vi "CALC_MARK_FUNC_SEL.vi"(0 "VISA IN":refnum<visa-resource-name>, 1 "Marker number":i32=1, 2 "Function":string(combo)="MAX", 5 "error in":errorcluster, 7 "Channel":i32=1) -> (14 "VISA Out":refnum<visa-resource-name>, 19 "error out":errorcluster)   [LabVIEW 2018, in "PNA-X.lvlib"]
doc: "CALCulate<cnum>:MARKer<mkr>:FUNCtion[:SELect] <char> \n(Read-Write) Sets the search function that the specified marker will perform when executed. To \nexecute (or perform) the function, use: \nCALC:MARK:FUNC:EXEC or \nCALC:MARK:FUNC:TRAC ON to automatically execute the search every sweep. \nSee Critical Note \nParameters \n<cnum> Channel number of the measurement. There must be a selected measurement on \nthat channel. If unspecified, <cnum> is set to 1. \n<mkr> Any marker number from 1 to 10; if unspecified, value is set to 1. \n<char> Marker function. Choose from: \nMAXimum - finds the highest value \nMINimum - finds the lowest value \nRPEak - finds the next valid peak to the right \nLPEak - finds the next valid peak to the left \nNPEak - finds the next highest value among the valid peaks \nTARGet - finds the target value to the right, wraps around to the left \nLTARget - finds the next target value to the left of the marker \nRTARget - finds the next target value to the right of the marker \nExamples CALC:MARK:FUNC MAX \ncalculate2:marker8:function:select ltarget \nQuery Syntax CALCulate<cnum>:MARKer<mkr>:FUNCtion[:SELect]? \nReturn Type Character \nDefault MAX \n1537"
uses:
  PNA-X.lvlib
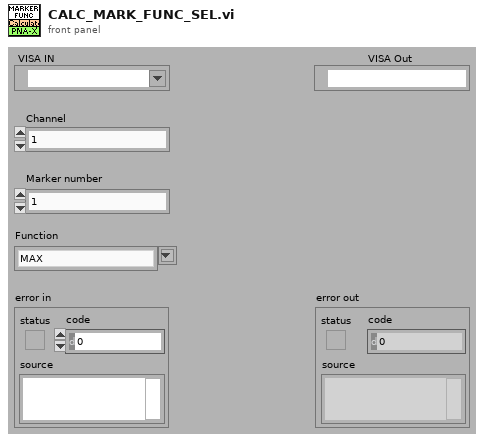
[diagram p1: front panel]
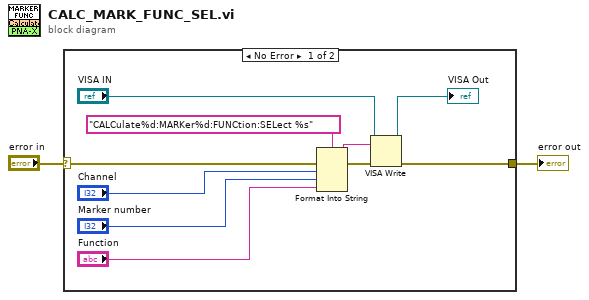
[diagram p0: block diagram]
diagram:
  n1 = case shown="No Error" "error in" {
    selector: "error in" -> [w12 w13]
    tunnel: [w7 w13] -> w1
    frame No Error {
      n2 = Format Into String(format string="CALCulate%d:MARKer%d:FUNCtion:SELect %s" ("Cmdline"), error in=w12, "Channel", "Marker number", "Function") -> (resulting string=w10:string, error out=w11:errorcluster)  [unwired: 1 in]
      n3 = VISA Write(VISA resource name="VISA IN", write buffer=w10, error in (no error)=w11) -> (VISA resource name out=→"VISA Out":refnum<visa-resource-name>, error out=w7:errorcluster)  [unwired: 1 out]
    }
    frame Error {
    }
  }
  "error out" <- w1
